vi "Fetch_PLCModbus InputIO.vi"(8 "error in (no error)":errorcluster, 9 "Status":bool, 10 "Insert":i32, 11 "Enum":T1) -> (0 "error out":errorcluster, 2 "Array":bool[](array[boolean]), 3 "Read":bool)   [LabVIEW 2019]
uses:
  Ctrl/123.ctl
panel:
  in  "Write PLCModbus Input":bool[](array[boolean])
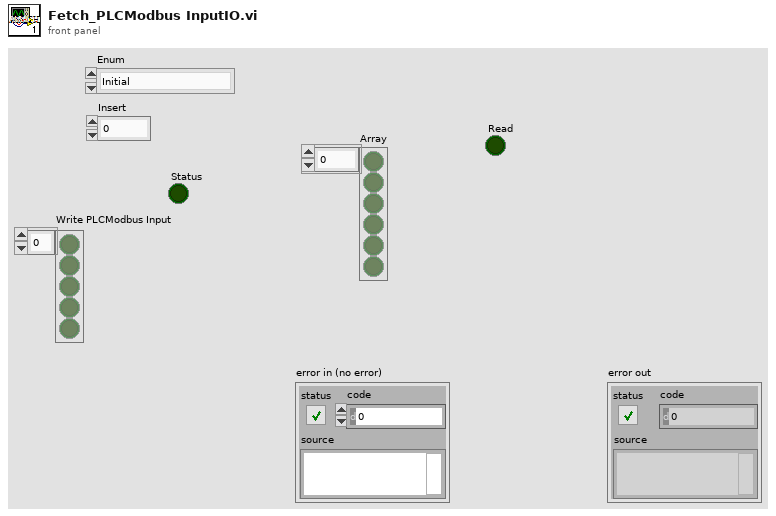
[diagram p1: front panel]
types:
  T1 = typedef "123.ctl" = enum16{"Initial", "Write", "Read"}
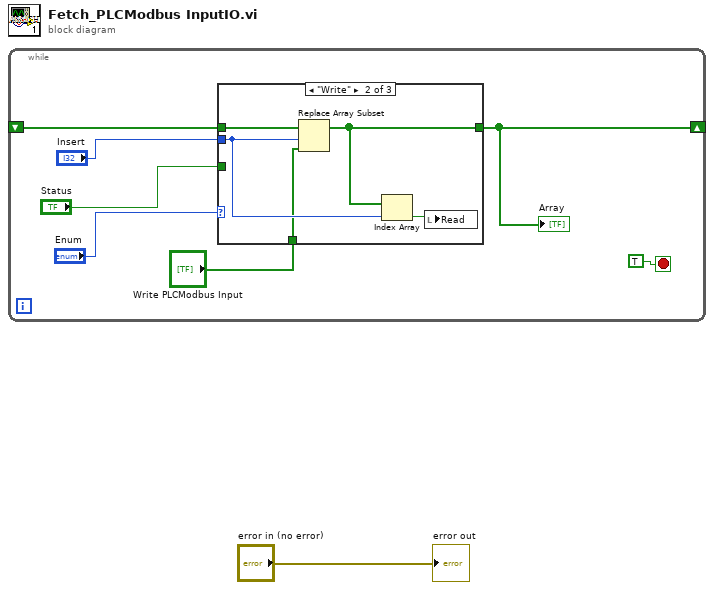
[diagram p0: block diagram]
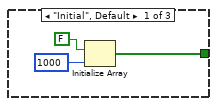
[diagram p2: hidden frame]
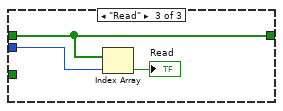
[diagram p3: hidden frame]
diagram:
  n1 = while {
    shift-right: [w4] -> _
    shift-left: _ -> [w7]
    stop <- TRUE stop-if-true
    n2 = case shown="\"Write\"" "Enum" {
      tunnel: w7 -> [_ w16 w19]
      tunnel: [w10 w14 w19] -> w4
      tunnel: "Insert" -> [_ w15 w18]
      tunnel: "Status" -> [_ _ _]
      tunnel: "Write PLCModbus Input" -> [_ w12 _]
      frame "Initial", Default {
        n3 = Initialize Array(FALSE, 1000 ("dimension size")) -> (w10:bool[])
      }
      frame "Write" {
        n4 = Replace Array Subset "Replace Array Subset"(array=w16, new element=w12, index=w15) -> (w14:bool[])
        n5 = Index Array(array=w14, index=w15) -> (element=w13:bool)
        n6 = local write "Read"(w13) -> ()
      }
      frame "Read" {
        n7 = Index Array(array=w19, index=w18) -> (element=→"Read":bool)
      }
    }
    "Array" <- w4
  }
  "error out" <- "error in (no error)"
